vi "white noise test.vi"   [LabVIEW 2018]
uses:
  <vilib>/DAQmx/write.llb/DAQmx Write (Analog DBL 1Chan 1Samp).vi
  <userlib>/DAQNavi Polymorphic VI/create/DAQNavi Create Channel(CI-UpDown Count Value).vi
  <userlib>/DAQNavi Polymorphic VI/read/DAQNavi Read (Counter Count Value 1Chan 1Samp).vi
  <vilib>/DAQmx/miscellaneous.llb/DAQmx Fill In Error Info.vi
  <vilib>/Analysis/NI_AALBase.lvlib
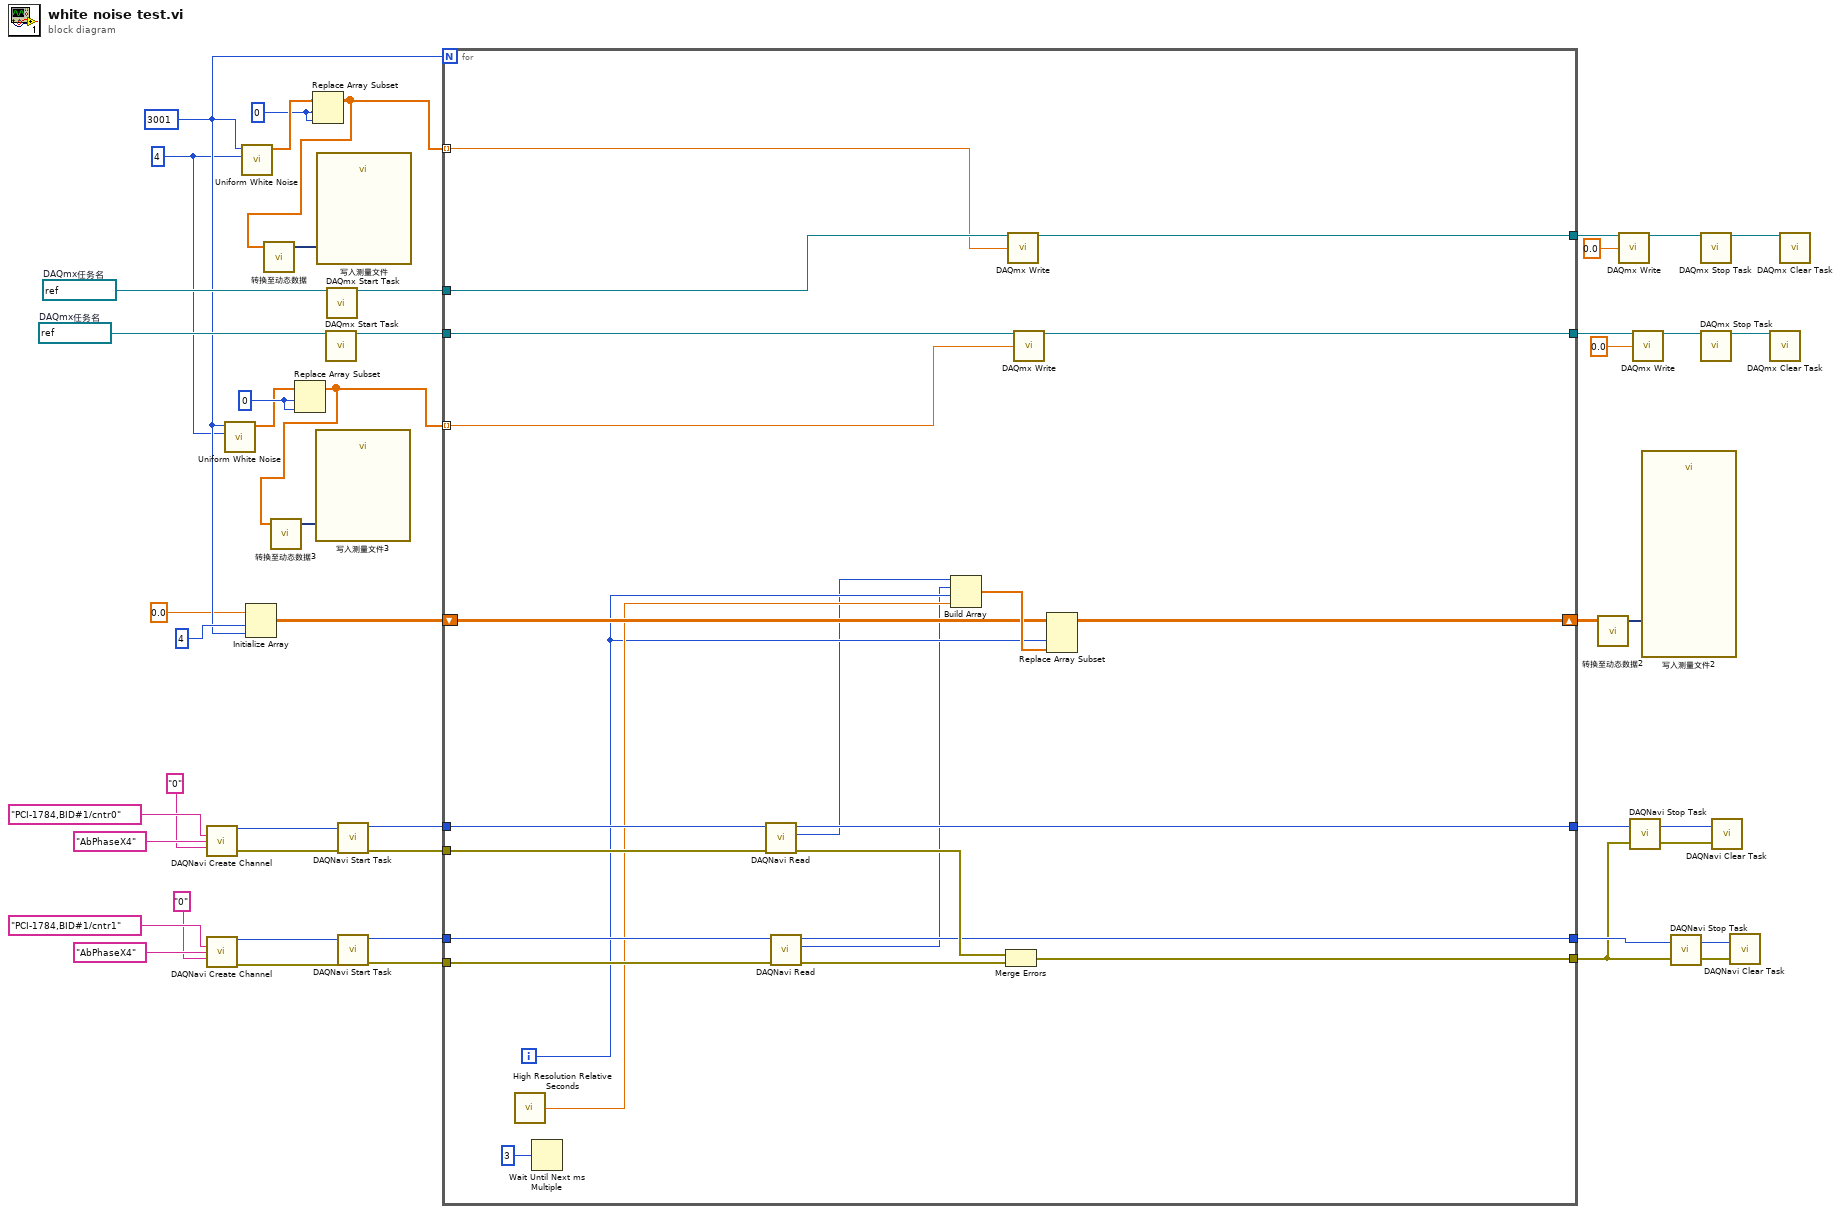
[diagram p0: block diagram]
diagram:
  w6 = 0
  w2 = 0
  w30 = 3001
  w29 = 4
  w47 = refnum<k21> "Stage_Y"  # DAQmx任务名
  w48 = refnum<k21> "Stage_X"  # DAQmx任务名
  n1 = call-poly <userlib>:"DAQNavi Create Channel.vi"("physical channels"="PCI-1784,BID#1/cntr0" ("Image Name"), "signal counting type"="AbPhaseX4" ("Image Name"), "initial value"="0" ("Image Name")) -> ("task out"=w23:i32, "error out"=w22:errorcluster)  [unwired: 11 in]
  n2 = call-poly <userlib>:"DAQNavi Create Channel.vi"("physical channels"="PCI-1784,BID#1/cntr1" ("Image Name"), "signal counting type"="AbPhaseX4" ("Image Name"), "initial value"="0" ("Image Name")) -> ("task out"=w21:i32, "error out"=w20:errorcluster)  [unwired: 11 in]
  n3 = call <vilib>:"Uniform White Noise.vi"("amplitude"=w29, "samples"=w30) -> ("uniform white noise"=w5:dbl[])  [unwired: 8 in, 1 out]
  n4 = call <vilib>:"Uniform White Noise.vi"("amplitude"=w29, "samples"=w30) -> ("uniform white noise"=w3:dbl[])  [unwired: 8 in, 1 out]
  n5 = Initialize Array(0.0, 4, w30) -> (w33:dbl[][])
  n6 = Replace Array Subset(array=w5, new element=w6, index=w6) -> (w4:dbl[])
  n7 = call "转换至动态数据3"("Array"=w4) -> ("Dynamic Data Type"=w31:dynamicdata)  [unwired: 3 in]
  n8 = Replace Array Subset(array=w3, new element=w2, index=w2) -> (w1:dbl[])
  n9 = call "转换至动态数据"("Array"=w1) -> ("Dynamic Data Type"=w36:dynamicdata)  [unwired: 3 in]
  n10 = call "写入测量文件3"("Signals"=w31) -> ()  [unwired: 16 in, 3 out]
  n11 = call "写入测量文件"("Signals"=w36) -> ()  [unwired: 16 in, 3 out]
  n12 = call <vilib>:"DAQmx Start Task.vi"("task/channels in"=w47) -> ("task out"=w45:refnum<k21>)  [unwired: 13 in, 1 out]
  n13 = call <vilib>:"DAQmx Start Task.vi"("task/channels in"=w48) -> ("task out"=w46:refnum<k21>)  [unwired: 13 in, 1 out]
  n14 = call <userlib>:"DAQNavi Start Task.vi"("error in (no error)"=w22, "task in"=w23) -> ("error out"=w17:errorcluster, "task out"=w16:i32)  [unwired: 8 in]
  n15 = call <userlib>:"DAQNavi Start Task.vi"("error in (no error)"=w20, "task in"=w21) -> ("error out"=w14:errorcluster, "task out"=w15:i32)  [unwired: 8 in]
  n16 = for {
    N: w30 -> [_]
    tunnel: w46 -> [w71]
    tunnel: w45 -> [w70]
    tunnel: [w69] -> w38
    tunnel: [w68] -> w37
    shift-right: [w64] -> w32
    shift-left: w33 -> [w65]
    tunnel: w4 -> [w53] mode=indexing
    tunnel: w1 -> [w63] mode=indexing
    tunnel: w17 -> [w60]
    tunnel: w16 -> [w59]
    tunnel: w15 -> [w58]
    tunnel: w14 -> [w57]
    tunnel: [w56] -> w9
    tunnel: [w55] -> w8
    tunnel: [w54] -> w7
    i -> [w51]
    n17 = call <vilib>:"High Resolution Relative Seconds.vi"() -> ("relative seconds"=w52:dbl)
    n18 = Wait Until Next ms Multiple(millisecond multiple=3) -> ()  [unwired: 1 out]
    n19 = call-poly <userlib>:"DAQNavi Read.vi"("error in (no error)"=w60, "task in"=w59) -> ("error out"=w61:errorcluster, "data"=w49:i32, "task out"=w56:i32)  [unwired: 7 in]
    n20 = call-poly <userlib>:"DAQNavi Read.vi"("error in (no error)"=w57, "task in"=w58) -> ("error out"=w62:errorcluster, "data"=w50:i32, "task out"=w55:i32)  [unwired: 7 in]
    n21 = Build Array(w49, w50, w51, w52) -> (w66:dbl[])
    n22 = Merge Errors(w61, w62) -> (w54:errorcluster)
    n23 = call-poly <vilib>:"DAQmx Write.vi"("task/channels in"=w71, "data"=w63) -> ("task out"=w69:refnum<k21>)  [unwired: 11 in, 2 out]
    n24 = call-poly <vilib>:"DAQmx Write.vi"("task/channels in"=w70, "data"=w53) -> ("task out"=w68:refnum<k21>)  [unwired: 11 in, 2 out]
    n25 = Replace Array Subset(array=w65, new element=w66, index (col)=w51) -> (w64:dbl[][])  [unwired: 1 in]
  }
  n26 = call "转换至动态数据2"("2D Array"=w32) -> ("Dynamic Data Type"=w35:dynamicdata)  [unwired: 3 in]
  n27 = call-poly <vilib>:"DAQmx Write.vi"("task/channels in"=w38, "data"=0.0) -> ("task out"=w44:refnum<k21>)  [unwired: 11 in, 2 out]
  n28 = call <userlib>:"DAQNavi Stop Task.vi"("error in (no error)"=w7, "task in"=w9) -> ("error out"=w12:errorcluster, "task out"=w13:i32)
  n29 = call-poly <vilib>:"DAQmx Write.vi"("task/channels in"=w37, "data"=0.0) -> ("task out"=w42:refnum<k21>)  [unwired: 11 in, 2 out]
  n30 = call "写入测量文件2"("Signals"=w35) -> ()  [unwired: 16 in, 3 out]
  n31 = call <userlib>:"DAQNavi Stop Task.vi"("error in (no error)"=w7, "task in"=w8) -> ("error out"=w10:errorcluster, "task out"=w11:i32)
  n32 = call <vilib>:"DAQmx Stop Task.vi"("task/channels in"=w44) -> ("task out"=w40:refnum<k21>)  [unwired: 13 in, 1 out]
  n33 = call <vilib>:"DAQmx Stop Task.vi"("task/channels in"=w42) -> ("task out"=w39:refnum<k21>)  [unwired: 13 in, 1 out]
  n34 = call <userlib>:"DAQNavi Clear Task.vi"("error in (no error)"=w12, "task in"=w13) -> ()  [unwired: 1 in, 1 out]
  n35 = call <userlib>:"DAQNavi Clear Task.vi"("error in (no error)"=w10, "task in"=w11) -> ()  [unwired: 1 in, 1 out]
  n36 = call <vilib>:"DAQmx Clear Task.vi"("task in"=w39) -> ()  [unwired: 14 in, 1 out]
  n37 = call <vilib>:"DAQmx Clear Task.vi"("task in"=w40) -> ()  [unwired: 14 in, 1 out]
